vi "Init_Values_for_power_kit_on Global.vi"(11 "DevSerialNum":string) -> (3 "JSON string":string)   [LabVIEW 2015]
uses:
  Share Data/uPower_kit.ctl
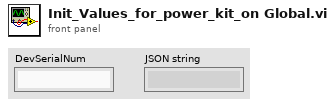
[diagram p1: front panel]
types:
  T1 = typedef "uPower_kit.ctl" = cluster{"DEV":string, "BUSY":bool, "VBAT":dbl, "OUTPUT":bool, "LAST_RESULT":dbl, "DURATION":u16, "TRIGGER":bool, "RANGE":string, "Vsource":dbl, "FW":string, "Mode":string}
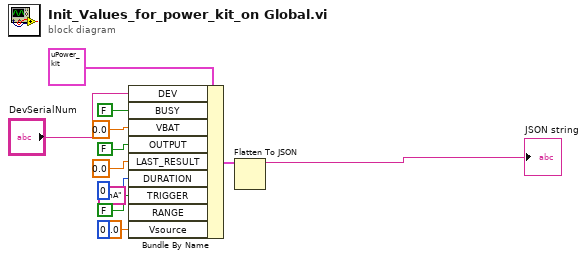
[diagram p0: block diagram]
diagram:
  (unwired) u8 0 ("RANGE")
  n1 = Bundle By Name(cluster=T1 {"DEV"="", "BUSY"=FALSE, "VBAT"=0.0, "OUTPUT"=FALSE, "LAST_RESULT"=0.0, "DURATION"=0, "TRIGGER"=FALSE, "RANGE"="", "Vsource"=0.0, "FW"="", "Mode"=""} ("DEV_BUSY"), "DEV"="DevSerialNum", "BUSY"=FALSE, "VBAT"=0.0, "OUTPUT"=FALSE, "LAST_RESULT"=0.0, "DURATION"=u16 0, "TRIGGER"=FALSE, "RANGE"="mA", "Vsource"=0.0) -> (w10:T1)
  n2 = Flatten To JSON(anything=w10) -> (JSON string=→"JSON string":string)  [unwired: 2 in, 1 out]
